vi "Execute.vi"(8 "error in":errorcluster, 11 "Wait STEP in":refnum<class "Wait STEP.lvclass">) -> (0 "error out":errorcluster, 1 "Next Step?":bool, 2 "MSG":string, 3 "Wait STEP out":refnum<class "Wait STEP.lvclass">)   [LabVIEW 2014, in "Calibration.lvlib" / "Wait STEP.lvclass"]
uses:
  Wait STEP.lvclass
  reusable/Sequence/STEPS/STEP.lvclass/STEP.ctl
  reusable/Sequence/STEPS/LEAVES/Double/Switch DBL.lvclass/Switch DBL.ctl
  reusable/Sequence/STEPS/Write First Call.vi
  reusable/Sequence/STEPS/Read First Call.vi
  reusable/Sequence/STEPS/LEAVES/Double/Read val.vi
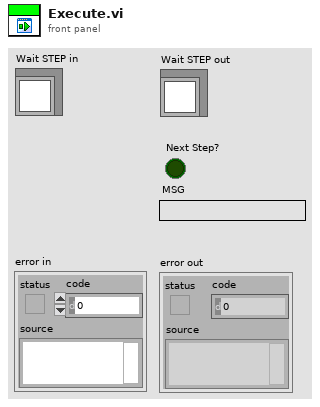
[diagram p1: front panel]
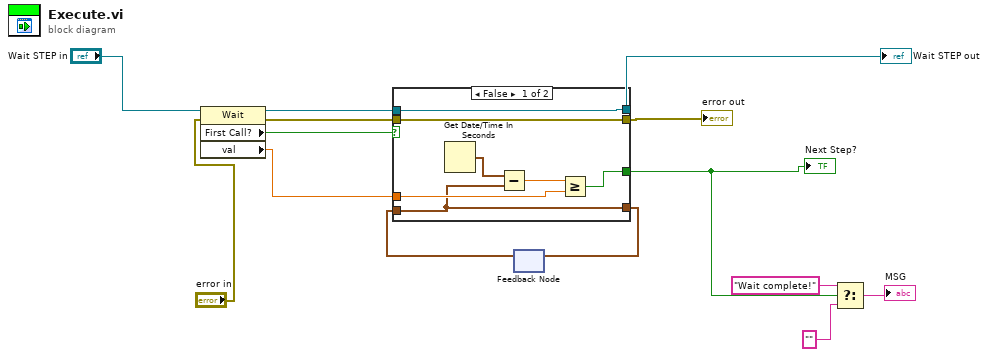
[diagram p0: block diagram]
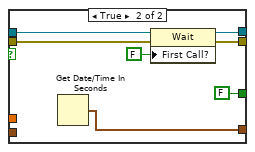
[diagram p2: hidden frame]
diagram:
  n1 = property class="Wait"(reference="Wait STEP in", error in="error in") -> (reference out=w12:refnum<class "Wait STEP.lvclass">, error out=w6:errorcluster, "First Call?"=w13:bool, "val"=w9:dbl)
  n2 = feedback #1() -> (w10:timestamp)  [unwired: 1 in]
  n3 = case shown="False" w13 {
    tunnel: w12 -> [w16 w28]
    tunnel: [w18 w26] -> w11
    tunnel: w10 -> [w18 _]
    tunnel: w9 -> [w19 _]
    tunnel: [w17 FALSE] -> w4
    tunnel: [w16 w24] -> w8
    tunnel: w6 -> [w15 w23]
    tunnel: [w15 w22] -> w5
    frame False {
      n4 = Get Date/Time In Seconds() -> (seconds since 1Jan1904=w21:timestamp)
      n5 = Subtract(x=w21, y=w18) -> (x-y=w20:dbl)
      n6 = Greater Or Equal?(x=w20, y=w19) -> (x >= y?=w17:bool)
    }
    frame True {
      n7 = Get Date/Time In Seconds() -> (seconds since 1Jan1904=w26:timestamp)
      n8 = property class="Wait"(reference=w28, error in=w23, "First Call?"=FALSE) -> (reference out=w24:refnum<class "Wait STEP.lvclass">, error out=w22:errorcluster)
    }
  }
  "error out" <- w5
  "Wait STEP out" <- w8
  "Next Step?" <- w4
  n9 = feedback-in #1(w11) -> ()
  n10 = Select(t="Wait complete!", s=w4, f="") -> (s? t:f=→"MSG":string)
